vi "worksheet set tab color.vi"(8 "error in (no error)":errorcluster, 10 "color":u32, 11 "worksheet":u32) -> (0 "error out":errorcluster)   [LabVIEW 8.6]
doc: "void worksheet_set_tab_color(lxw_worksheet worksheet, lxw_color_t color);"
uses:
  pending_lvxlsxwriter/xlsxwriter.dll
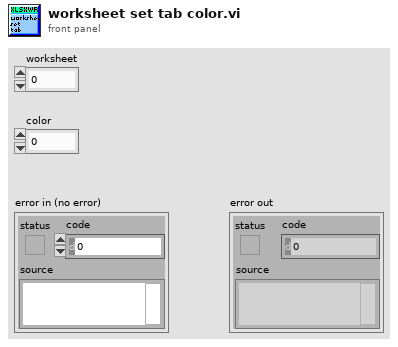
[diagram p1: front panel]
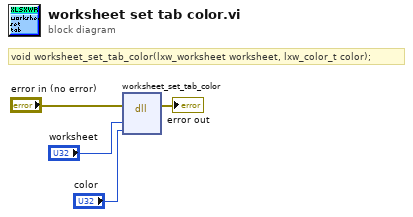
[diagram p0: block diagram]
diagram:
  # "void worksheet_set_tab_color(lxw_worksheet worksheet, lxw_color_t color);"
  n1 = dll-call lib="C:/Users/WDAGUtilityAccount/Desktop/pending_lvxlsxwriter/xlsxwriter.*" fn="worksheet_set_tab_color"(error in="error in (no error)", "worksheet"="worksheet", "color"="color") -> (error out=→"error out":errorcluster)  [unwired: 5 in, 1 out]
